vi "Turn Motors Off.vi"   [LabVIEW 2009]
uses:
  Motor Output Global.vi
  <vilib>/eio/EIONode/EIONode.xnode
  <vilib>/rvi/eio/nirviEIOImplementation/nirviEIOImplementation.xnode
  <vilib>/rvi/eio/common/nirviEmuTemplateMethod_noerrors.vi
  <vilib>/rvi/eio/common/nirviEmuClasses.ctl
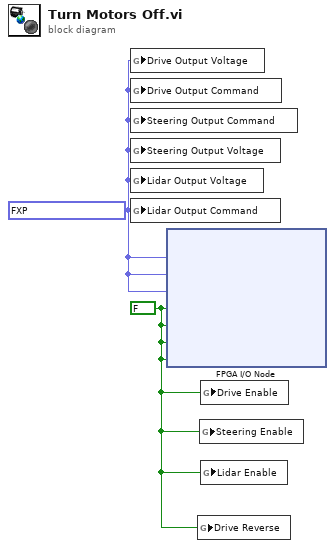
[diagram p0: block diagram]
diagram:
  w1 = fxp<+/-,20,5> 0.0 ("Steering output Voltage")
  w2 = FALSE ("stop")
  n1 = global write "Motor Output Global.vi" "Drive Output Voltage"(w1) -> ()
  n2 = global write "Motor Output Global.vi" "Drive Output Command"(w1) -> ()
  n3 = global write "Motor Output Global.vi" "Steering Output Command"(w1) -> ()
  n4 = global write "Motor Output Global.vi" "Steering Output Voltage"(w1) -> ()
  n5 = global write "Motor Output Global.vi" "Lidar Output Voltage"(w1) -> ()
  n6 = global write "Motor Output Global.vi" "Lidar Output Command"(w1) -> ()
  n7 = xnode "FPGA I/O Node"("Drive Motor Speed"=w1, "Steering Motor Speed"=w1, "Lidar Motor Speed"=w1, "Drive Motor Reverse"=w2, "Drive Motor Enable"=w2, "Steering Motor Inhibit"=w2, "Lidar Motor Inhibit"=w2) -> ()  [unwired: 7 in, 7 out]
  n8 = global write "Motor Output Global.vi" "Drive Reverse"(w2) -> ()
  n9 = global write "Motor Output Global.vi" "Steering Enable"(w2) -> ()
  n10 = global write "Motor Output Global.vi" "Drive Enable"(w2) -> ()
  n11 = global write "Motor Output Global.vi" "Lidar Enable"(w2) -> ()
